vi "제목없음 3.vi"() -> ()   [LabVIEW 2014]
panel:
  out "시간 측정":u32
  in  "정지":bool
  in  "확인 버튼":bool
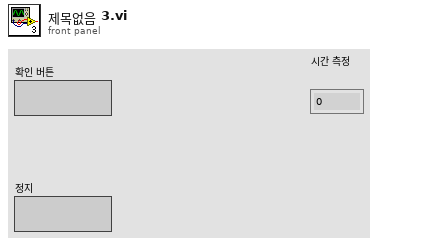
[diagram p1: front panel]
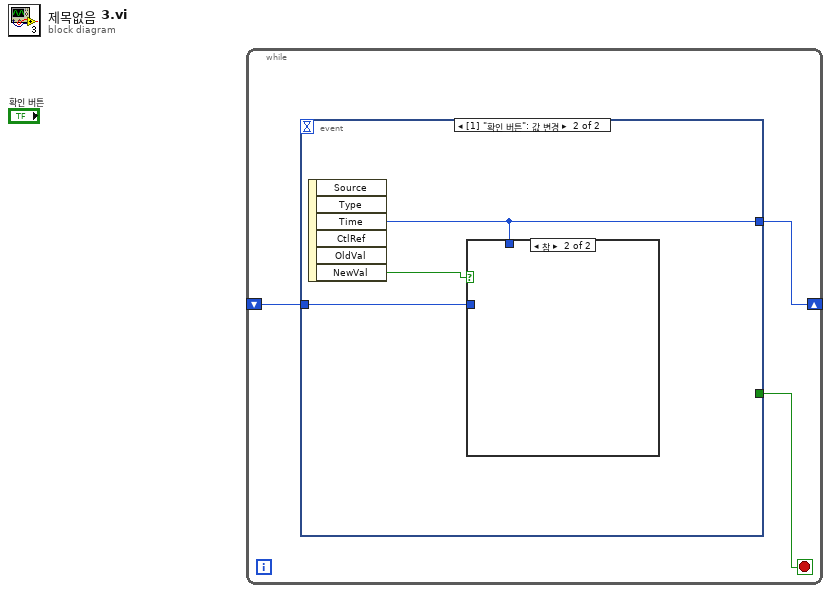
[diagram p0: block diagram]
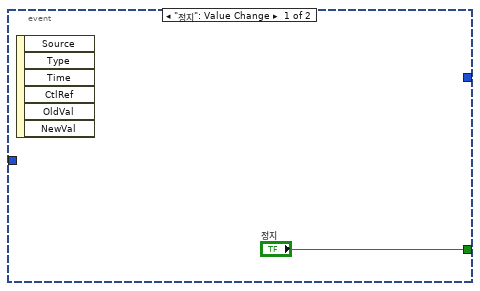
[diagram p2: hidden frame]
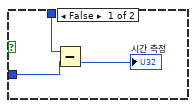
[diagram p3: hidden frame]
diagram:
  n1 = while {
    shift-right: [w2] -> _
    shift-left: _ -> [w1]
    stop <- w3 stop-if-true
    n2 = event shown="[1] \"확인 버튼\": 값 변경" {
      selector: _ -> [_ _]
      dyn-events: _ -> [_ _]
      timeout: _ -> [_ _]
      tunnel: ["정지" _] -> w3
      tunnel: [_ w6] -> w2
      tunnel: w1 -> [_ w5]
      event "정지": Value Change {
        n3 = event-data() -> ()  [unwired: 1 in, 6 out]
      }
      event "확인 버튼": Value Change {
        n4 = event-data() -> ("Time"=w6:u32, "NewVal"=w7:bool)  [unwired: 1 in, 4 out]
        n5 = case shown="참" w7 {
          tunnel: w6 -> [w10 _]
          tunnel: w5 -> [w9 _]
          frame False {
            n6 = Subtract(x=w10, y=w9) -> (x-y=→"시간 측정":u32)
          }
          frame True {
          }
        }
      }
    }
  }
